vi "Update position.vi"(0 "R pos":dbl[](array[numeric]), 1 "R dir":dbl(slide) scale=3.2..-3.2, 2 "dt":dbl, 3 "v":dbl, 4 "w":dbl) -> (5 "R pos new":dbl[](array[numeric]), 6 "R dir new":dbl(slide) scale=3.2..-3.2)   [LabVIEW 2009]
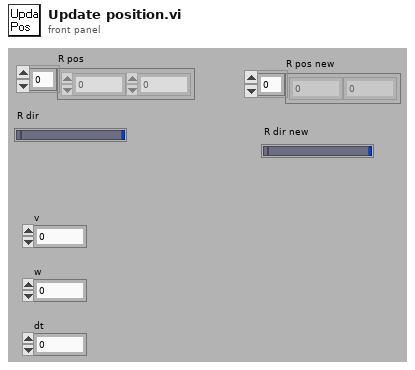
[diagram p1: front panel]
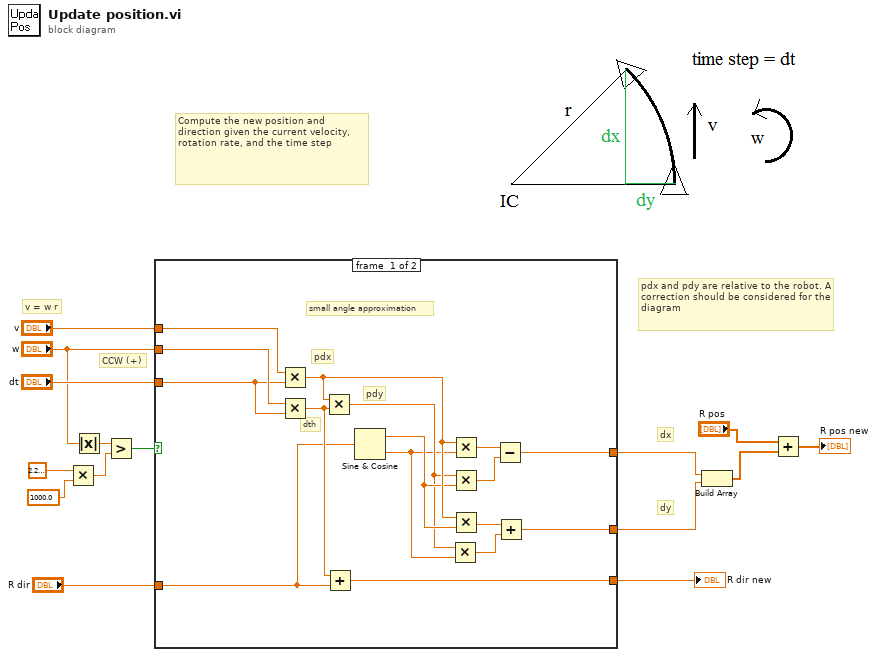
[diagram p0: block diagram]
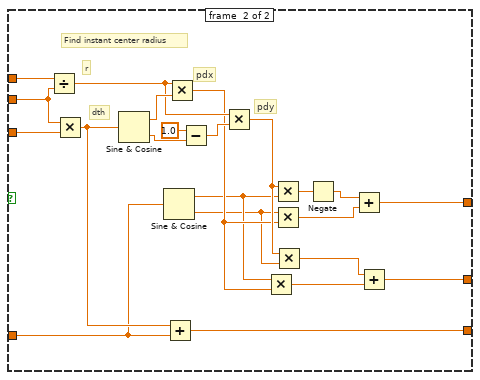
[diagram p2: hidden frame]
diagram:
  # "pdx and pdy are relative to the robot. A correction should be considered for the diagram"
  # "Compute the new position and direction given the current velocity, rotation rate, and the time step"
  # "dy"
  # "dx"
  # "CCW (+)"
  # "v = w r"
  n1 = Multiply(x=2.220446049250313e-16, y=1000.0) -> (x*y=w1:dbl)
  n2 = Absolute Value(x="w") -> (abs(x)=w5:dbl)
  n3 = Greater?(x=w5, y=w1) -> (0:w4:bool)
  n4 = case shown="True" w4 {
    tunnel: "v" -> [w31 w53]
    tunnel: "w" -> [w30 w52]
    tunnel: "dt" -> [w29 w51]
    tunnel: [w27 w50] -> w13
    tunnel: "R dir" -> [w26 w43]
    tunnel: [w23 w33] -> w11
    tunnel: [w16 w32] -> w10
    frame #0 {
      # "pdy"
      # "pdx"
      # "small angle approximation"
      # "dth"
      n5 = Multiply(x=w31, y=w29) -> (x*y=w22:dbl)
      n6 = Multiply(x=w30, y=w29) -> (x*y=w28:dbl)
      n7 = Multiply(x=w22, y=w28) -> (x*y=w18:dbl)
      n8 = Add(x=w28, y=w26) -> (x+y=w27:dbl)
      n9 = Sine & Cosine(0:w26) -> (1:w21:dbl, 2:w17:dbl)
      n10 = Multiply(x=w18, y=w17) -> (x*y=w19:dbl)
      n11 = Multiply(x=w22, y=w17) -> (x*y=w25:dbl)
      n12 = Multiply(x=w18, y=w21) -> (x*y=w24:dbl)
      n13 = Multiply(x=w22, y=w21) -> (x*y=w20:dbl)
      n14 = Subtract(x=w25, y=w24) -> (x-y=w23:dbl)
      n15 = Add(x=w20, y=w19) -> (x+y=w16:dbl)
    }
    frame #1 {
      # "pdy"
      # "pdx"
      # "dth"
      # "r"
      # "Find instant center radius"
      n16 = Divide(x=w53, y=w52) -> (x/y=w44:dbl)
      n17 = Multiply(x=w52, y=w51) -> (x*y=w49:dbl)
      n18 = Sine & Cosine(0:w49) -> (1:w46:dbl, 2:w48:dbl)
      n19 = Sine & Cosine(0:w43) -> (1:w37:dbl, 2:w36:dbl)
      n20 = Add(x=w49, y=w43) -> (x+y=w50:dbl)
      n21 = Multiply(x=w44, y=w46) -> (x*y=w38:dbl)
      n22 = Subtract(x=1.0, y=w48) -> (x-y=w45:dbl)
      n23 = Multiply(x=w44, y=w45) -> (x*y=w39:dbl)
      n24 = Multiply(x=w37, y=w38) -> (x*y=w34:dbl)
      n25 = Multiply(x=w39, y=w37) -> (x*y=w42:dbl)
      n26 = Multiply(x=w36, y=w38) -> (x*y=w40:dbl)
      n27 = Multiply(x=w39, y=w36) -> (x*y=w35:dbl)
      n28 = Negate(x=w42) -> (-x=w41:dbl)
      n29 = Add(x=w41, y=w40) -> (x+y=w33:dbl)
      n30 = Add(x=w35, y=w34) -> (x+y=w32:dbl)
    }
  }
  "R dir new" <- w13
  n31 = Build Array(w11, w10) -> (w8:dbl[])
  n32 = Add(x="R pos", y=w8) -> (x+y=→"R pos new":dbl[])
